vi "PoseAndTargeting.vi"() -> ()   [LabVIEW 2019]
doc: "This VI manages the robot's pose and targetting information. Data from the IMU, swerve drive encoders, swerve azimuth encoders, LimeLight, and LIDAR are fused together to estimate these values. Supports pose resets on boot, from the Autonomous Sequencer, and on command from the FRC 4265 Dashboard."
uses:
  dsinstructions.vi
  sensors.vi
  dsdata.vi
  outputs.vi
panel:
  out "Y Position (in)":dbl=94.7
  out "X Position (in)":dbl=509.2
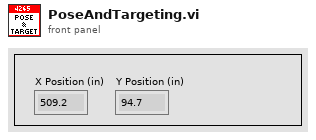
[diagram p1: front panel]
types:
  T1 = enum16{"Center", "North", "NorthWest", "West", "SouthWest", "South", "SouthEast", "East", "NorthEast"}
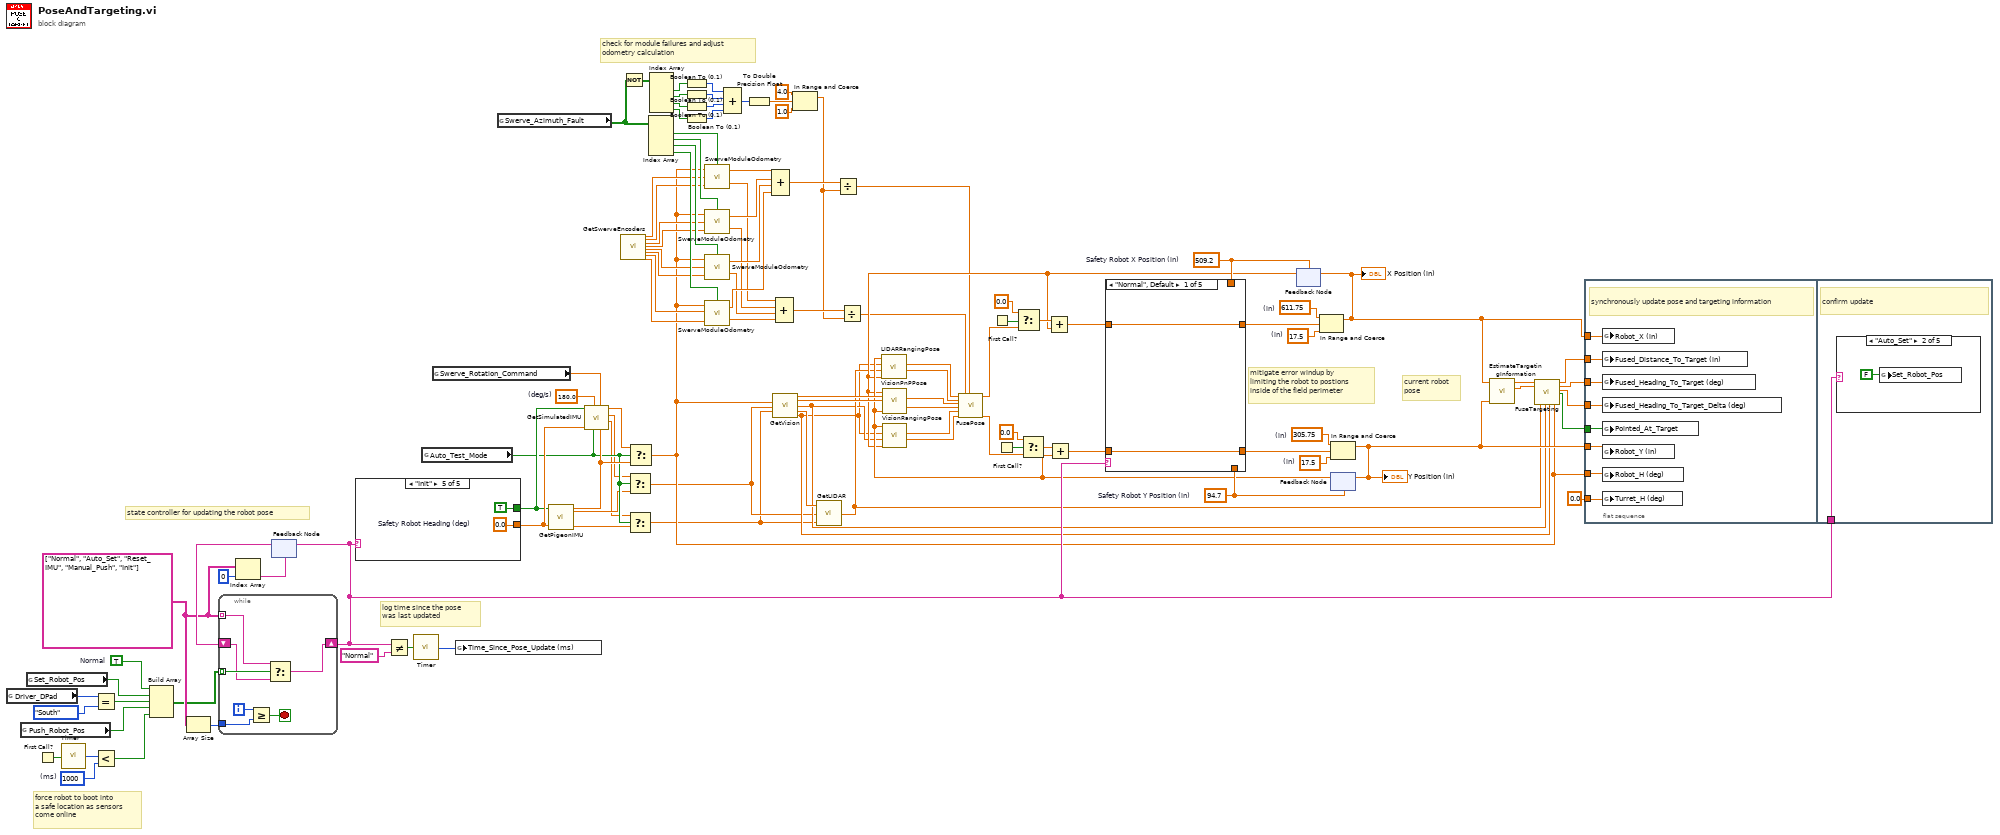
[diagram p0: block diagram]
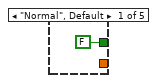
[diagram p6: hidden frame]
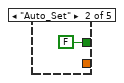
[diagram p7: hidden frame]
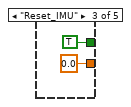
[diagram p8: hidden frame]
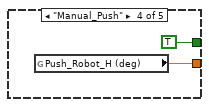
[diagram p9: hidden frame]
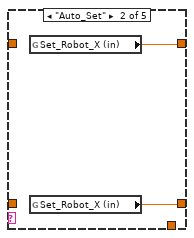
[diagram p10: hidden frame]
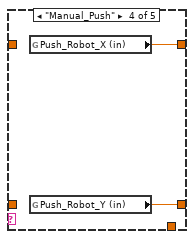
[diagram p12: hidden frame]
diagram:
  w50 = 180.0  # (deg/s)
  w54 = u32 1000  # (ms)
  w72 = string[] ["Normal", "Auto_Set", "Reset_IMU", "Manual_Push", "Init"] ("State Names")
  w71 = TRUE  # Normal
  w81 = 305.75  # (in)
  w82 = 17.5  # (in)
  w86 = 611.75  # (in)
  w87 = 17.5  # (in)
  w59 = 509.2  # Safety Robot X Position (in)
  w58 = 94.7  # Safety Robot Y Position (in)
  # "force robot to boot into\na safe location as sensors\ncome online"
  # "log time since the pose\nwas last updated"
  # "state controller for updating the robot pose"
  # "current robot\npose"
  # "mitigate error windup by\nlimiting the robot to postions\ninside of the field perimeter"
  # "check for module failures and adjust\nodometry calculation"
  n1 = global read "dsinstructions.vi" "Driver_DPad"() -> (w89:T1)
  n2 = global read "sensors.vi" "Push_Robot_Pos"() -> (w73:bool)
  n3 = global read "sensors.vi" "Set_Robot_Pos"() -> (w49:bool)
  n4 = First Call?() -> (First Call?: T/F=w57:bool)
  n5 = call "Timer.vi"("Reset Timer"=w57) -> ("Time (ms)"=w56:u32)
  n6 = Equal?(x=w89, y=T1."South") -> (x = y?=w48:bool)
  n7 = Less?(x=w56, y=w54) -> (x < y?=w55:bool)
  n8 = Build Array(w71, w49, w48, w73, w55) -> (w70:bool[])
  n9 = Array Size(array=w72) -> (size(s)=w74:i32)
  n10 = Index Array(array=w72, index=0) -> (element=w76:string)
  n11 = feedback #1(w76) -> (w75:string)
  n12 = while {
    tunnel: w70 -> [w121] mode=indexing
    tunnel: w72 -> [w119] mode=indexing
    shift-right: [w118] -> w63
    shift-left: w75 -> [w120]
    tunnel: w74 -> [w116]
    i -> [w117]
    stop <- w115 stop-if-true
    n13 = Greater Or Equal?(x=w117, y=w116) -> (x >= y?=w115:bool)
    n14 = Select(t=w119, s=w121, f=w120) -> (s? t:f=w118:string)
  }
  n15 = feedback-in #1(w63) -> ()
  n16 = case shown="\"Init\"" w63 {
    tunnel: [_ _ 0.0 ("Push_Robot_H (deg)") w127 w128] -> w53
    tunnel: [FALSE FALSE TRUE TRUE TRUE] -> w52
    frame "Normal", Default {
    }
    frame "Auto_Set" {
    }
    frame "Reset_IMU" {
    }
    frame "Manual_Push" {
      n17 = global read "sensors.vi" "Push_Robot_H (deg)"() -> (w127:dbl)
    }
    frame "Init" {
      w128 = 0.0  # Safety Robot Heading (deg)
    }
  }
  n18 = Not Equal?(x=w63, y="Normal") -> (x != y?=w62:bool)
  n19 = call "Timer.vi"("Reset Timer"=w62) -> ("Time (ms)"=w60:u32)
  n20 = global read "dsdata.vi" "Auto_Test_Mode"() -> (w8:bool)
  n21 = global read "outputs.vi" "Swerve_Rotation_Command"() -> (w51:dbl)
  n22 = global write "sensors.vi" "Time_Since_Pose_Update (ms)"(w60) -> ()
  n23 = global read "sensors.vi" "Swerve_Azimuth_Fault"() -> (w104:bool[])
  n24 = call "GetPigeonIMU.vi"("Reset Yaw (deg)"=w53, "Reset Yaw"=w52) -> ("Roll (deg)"=w4:dbl, "Pitch (deg)"=w6:dbl, "Yaw (deg)"=w9:dbl)  [unwired: 7 in]
  n25 = call "GetSimulatedIMU.vi"("Real IMU Yaw (deg)"=w9, "Rotation Command"=w51, "Auto Test Mode"=w8, "Max Simulated Rotation Speed (deg/s)"=w50, "Reset Yaw (deg)"=w53, "Reset Yaw"=w52) -> ("Simulated Roll (deg)"=w5:dbl, "Simulated Pitch (deg)"=w7:dbl, "Simulated Yaw (deg)"=w10:dbl)  [unwired: 3 in]
  n26 = call "GetSwerveEncoders.vi"() -> ("Swerve 0 Azimuth Position (deg)"=w47:dbl, "Swerve 0 Distance (in)"=w40:dbl, "Swerve 1 Azimuth Position (deg)"=w46:dbl, "Swerve 1 Distance (in)"=w45:dbl, "Swerve 2 Azimuth Position (deg)"=w44:dbl, "Swerve 2 Distance (in)"=w43:dbl, "Swerve 3 Azimuth Position (deg)"=w42:dbl, "Swerve 3 Distance (in)"=w41:dbl)  [unwired: 20 in]
  n27 = Not(x=w104) -> (.not. x?=w103:bool[])
  n28 = Select(t=w7, s=w8, f=w6) -> (s? t:f=w2:dbl)
  n29 = Select(t=w5, s=w8, f=w4) -> (s? t:f=w1:dbl)
  n30 = Select(t=w10, s=w8, f=w9) -> (s? t:f=w3:dbl)
  n31 = Index Array(array=w104) -> (element #1=w93:bool, element #2=w92:bool, element #3=w91:bool, element #4=w90:bool)  [unwired: 4 in]
  n32 = Index Array(array=w103) -> (element #1=w102:bool, element #2=w101:bool, element #3=w100:bool, element #4=w99:bool)  [unwired: 4 in]
  n33 = Boolean To (0,1)(Boolean=w102) -> (0, 1=w98:i16)
  n34 = Boolean To (0,1)(Boolean=w101) -> (0, 1=w97:i16)
  n35 = Boolean To (0,1)(Boolean=w100) -> (0, 1=w96:i16)
  n36 = Boolean To (0,1)(Boolean=w99) -> (0, 1=w95:i16)
  n37 = call "SwerveModuleOdometry.vi"("Module Fault"=w93, "Wheel Distance (in)"=w40, "Wheel Azimuth (deg)"=w47, "Robot Heading(deg)"=w3) -> ("Delta Y (in)"=w105:dbl, "Delta X (in)"=w114:dbl)
  n38 = call "SwerveModuleOdometry.vi"("Module Fault"=w92, "Wheel Distance (in)"=w45, "Wheel Azimuth (deg)"=w46, "Robot Heading(deg)"=w3) -> ("Delta Y (in)"=w106:dbl, "Delta X (in)"=w113:dbl)
  n39 = call "SwerveModuleOdometry.vi"("Module Fault"=w91, "Wheel Distance (in)"=w43, "Wheel Azimuth (deg)"=w44, "Robot Heading(deg)"=w3) -> ("Delta Y (in)"=w107:dbl, "Delta X (in)"=w112:dbl)
  n40 = call "SwerveModuleOdometry.vi"("Module Fault"=w90, "Wheel Distance (in)"=w41, "Wheel Azimuth (deg)"=w42, "Robot Heading(deg)"=w3) -> ("Delta Y (in)"=w108:dbl, "Delta X (in)"=w111:dbl)
  n41 = Compound Arithmetic op=ADD(w98, w97, w96, w95) -> (w94:i16)
  n42 = To Double Precision Float(number=w94) -> (double precision float=w35:dbl)
  n43 = Compound Arithmetic op=ADD(w114, w113, w112, w111) -> (w110:dbl)
  n44 = call "GetVision.vi"("Robot_H (deg)"=w3, "Pitch (deg)"=w2, "Roll (deg)"=w1) -> ("LimeLight Raw Z (in)"=w39:dbl, "LimeLight Raw X (in)"=w38:dbl, "LimeLight Distance to Target (in)"=w17:dbl, "LimeLight Raw Horizontal Offset (deg)"=w19:dbl, "LimeLight Heading to Target (deg)"=w12:dbl)  [unwired: 8 in]
  n45 = Compound Arithmetic op=ADD(w105, w106, w107, w108) -> (w109:dbl)
  n46 = In Range and Coerce(upper limit=4.0, x=w35, lower limit=1.0) -> (coerced(x)=w32:dbl)  [unwired: 1 out]
  n47 = call "GetLIDAR.vi"("Roll (deg)"=w1, "Pitch (deg)"=w2, "Raw Horizontal Offset (in)"=w19) -> ("LIDAR Distance to Target (in)"=w18:dbl)
  n48 = Divide(x=w110, y=w32) -> (x/y=w29:dbl)
  n49 = Divide(x=w109, y=w32) -> (x/y=w28:dbl)
  n50 = First Call?() -> (First Call?: T/F=w84:bool)
  n51 = First Call?() -> (First Call?: T/F=w79:bool)
  n52 = feedback #2(w59) -> (w36:dbl)
  n53 = feedback #3(w58) -> (w37:dbl)
  n54 = call "LIDARRangingPose.vi"("Previous X Position (in)"=w36, "Distance to Target (in)"=w18, "Heading to Target (deg)"=w12, "Previous Y Position (in)"=w37) -> ("Delta Y (in)"=w26:dbl, "Delta X (in)"=w27:dbl)  [unwired: 6 in]
  n55 = call "VisionPnPPose.vi"("Previous Y Estimate (in)"=w37, "LimeLight Raw X (in)"=w38, "LimeLight Raw Z (in)"=w39, "Previous X Estimate (in)"=w36) -> ("deltaY (in)"=w24:dbl, "deltaX (in)"=w25:dbl)  [unwired: 6 in]
  n56 = call "VisionRangingPose.vi"("Previous X Position (in)"=w36, "Distance to Target (in)"=w17, "Heading to Target (deg)"=w12, "Previous Y Position (in)"=w37) -> ("Delta Y (in)"=w22:dbl, "Delta X (in)"=w23:dbl)  [unwired: 6 in]
  n57 = call "FusePose.vi"("LIDAR range deltaX"=w27, "LIDAR range deltaY"=w26, "LimeLight PnP deltaX"=w25, "LimeLight PnP deltaY"=w24, "LimeLight range deltaX"=w23, "LimeLight range deltaY"=w22, "Odometry deltaY"=w28, "Odometry deltaX"=w29) -> ("Fused deltaX"=w31:dbl, "Fused deltaY"=w30:dbl)  [unwired: 10 in]
  n58 = Select(t=0.0, s=w84, f=w31) -> (s? t:f=w85:dbl)
  n59 = Select(t=0.0, s=w79, f=w30) -> (s? t:f=w80:dbl)
  n60 = Add(x=w85, y=w36) -> (x+y=w69:dbl)
  n61 = Add(x=w80, y=w37) -> (x+y=w67:dbl)
  n62 = case shown="\"Normal\", Default" w63 {
    tunnel: w69 -> [w131 _ w135 _ _]
    tunnel: [w131 w133 w135 w137 w139] -> w68
    tunnel: w67 -> [w130 _ w134 _ _]
    tunnel: [w130 w132 w134 w136 w138] -> w66
    tunnel: w59 -> [_ _ _ _ w139]
    tunnel: w58 -> [_ _ _ _ w138]
    frame "Normal", Default {
    }
    frame "Auto_Set" {
      n63 = global read "sensors.vi" "Set_Robot_X (in)"() -> (w133:dbl)
      n64 = global read "sensors.vi" "Set_Robot_X (in)"() -> (w132:dbl)
    }
    frame "Reset_IMU" {
    }
    frame "Manual_Push" {
      n65 = global read "sensors.vi" "Push_Robot_X (in)"() -> (w137:dbl)
      n66 = global read "sensors.vi" "Push_Robot_Y (in)"() -> (w136:dbl)
    }
    frame "Init" {
    }
  }
  n67 = In Range and Coerce(upper limit=w86, x=w68, lower limit=w87) -> (coerced(x)=w65:dbl)  [unwired: 1 out]
  "X Position (in)" <- w65
  n68 = feedback-in #2(w65) -> ()
  n69 = In Range and Coerce(upper limit=w81, x=w66, lower limit=w82) -> (coerced(x)=w64:dbl)  [unwired: 1 out]
  "Y Position (in)" <- w64
  n70 = feedback-in #3(w64) -> ()
  n71 = call "EstimateTargetingInformation.vi"("Robot Y (in)"=w64, "Robot X (in)"=w65) -> ("Estimated Robot Heading to Target (deg)"=w20:dbl, "Estimated Distance to Target (in)"=w21:dbl)  [unwired: 7 in]
  n72 = call "FuseTargeting.vi"("Estimated Distance to Target (in)"=w21, "Estimated Heading to Target (deg)"=w20, "LIDAR Distance to Target (in)"=w18, "LimeLight Distance to Target (in)"=w17, "LimeLight Heading to Target (deg)"=w12, "Robot_H (deg)"=w3) -> ("Fused Distance to Target (in)"=w16:dbl, "Fused Heading to Target (deg)"=w15:dbl, "Fused Heading to Target Delta (deg)"=w14:dbl, "Pointed at Target"=w13:bool)  [unwired: 10 in]
  n73 = flat-sequence {
    tunnel: w65 -> [w147]
    tunnel: w64 -> [w146]
    tunnel: w3 -> [w145]
    tunnel: w16 -> [w144]
    tunnel: w15 -> [w143]
    tunnel: w14 -> [w142]
    tunnel: w13 -> [w141]
    tunnel: 0.0 ("Turret_H (deg)") -> [w140]
    tunnel: w63 -> [w148]
    frame #0 {
      # "synchronously update pose and targeting information"
      n74 = global write "sensors.vi" "Robot_X (in)"(w147) -> ()
      n75 = global write "sensors.vi" "Fused_Distance_To_Target (in)"(w144) -> ()
      n76 = global write "sensors.vi" "Fused_Heading_To_Target (deg)"(w143) -> ()
      n77 = global write "sensors.vi" "Fused_Heading_To_Target_Delta (deg)"(w142) -> ()
      n78 = global write "sensors.vi" "Pointed_At_Target"(w141) -> ()
      n79 = global write "sensors.vi" "Robot_Y (in)"(w146) -> ()
      n80 = global write "sensors.vi" "Robot_H (deg)"(w145) -> ()
      n81 = global write "sensors.vi" "Turret_H (deg)"(w140) -> ()
    }
    frame #1 {
      # "confirm update"
      n82 = case shown="\"Auto_Set\"" w148 {
        frame "Normal", Default {
        }
        frame "Auto_Set" {
          n83 = global write "sensors.vi" "Set_Robot_Pos"(FALSE ("Set_Robot_Pos")) -> ()
        }
        frame "Reset_IMU" {
        }
        frame "Manual_Push" {
        }
        frame "Init" {
        }
      }
    }
  }
